vi "Write Origin.vi"(8 "error in (no error)":errorcluster, 10 "Origin":T1, 11 "SwipeMenu in":refnum<class "SwipeMenu.lvclass">) -> (0 "error out":errorcluster, 3 "SwipeMenu out":refnum<class "SwipeMenu.lvclass">)   [LabVIEW 2019, in "SwipeMenu.lvclass"]
uses:
  SwipeMenu.lvclass
  <vilib>/Utility/miscctls.llb/LVPointTypeDef.ctl
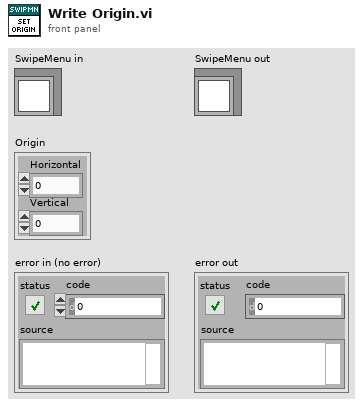
[diagram p1: front panel]
types:
  T1 = typedef "LVPointTypeDef.ctl" = cluster{"Horizontal":i16, "Vertical":i16}
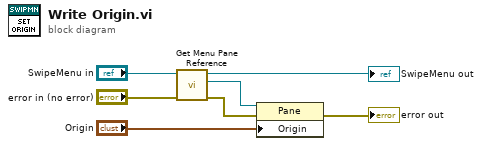
[diagram p0: block diagram]
diagram:
  n1 = call "Get Menu Pane Reference.vi"("error in (no error)"="error in (no error)", "SwipeMenu in"="SwipeMenu in") -> ("error out"=w1:errorcluster, "Menu Pane Refnum"=w2:refnum<vi>, "SwipeMenu out"=→"SwipeMenu out":refnum<class "SwipeMenu.lvclass">)  [unwired: 7 in]
  n2 = property class="Pane"(reference=w2, error in=w1, "Origin"="Origin") -> (error out=→"error out":errorcluster)  [unwired: 1 out]
